vi "PID_controller_16.vi"() -> ()   [LabVIEW 2011]
panel:
  in  "Ring":u16(ring)=2 items=["A", "B", "C", "D"]
  out "do_tune":bool
  in  "Tune":bool
  out "Tune Set Point (torr)":dbl
  in  "stop":bool
  out "fit":cluster{"element":dbl, "Value":dbl}[](array[cluster])
  out "err_avg":dbl
  out "Setpoint":string
  in  "Ks":dbl
  out "dt(s)":dbl
  out "windup error":dbl
  out "tPrev":dbl
  out "target value":dbl
  out "error(t-t0)":cluster{dbl, "Value":dbl}[](array[cluster])
  out "error":dbl
  out "tStart(s)":dbl
  out "S00":dbl
  out "S10":dbl
  out "S20":dbl
  out "S11":dbl
  out "S01":dbl
  out "weight":dbl[](array[numeric])
  in  "# of points to watch":i32=60
  in  "tSmooth(s)":dbl=4.0
  out "t0":dbl
  out "error(t)":cluster{dbl, "Value":dbl}[](array[cluster])
  out "error out":errorcluster
  out "first":bool=TRUE
  out "XY Graph":T1(graph)
  out "current value":dbl
  in  "Period (s)":dbl=1.0
  out "dValue":dbl
  out "derivative":dbl
  out "integral":dbl
  out "Angle (deg)":dbl
  in  "Kd":dbl=0.4
  in  "Ki":dbl
  in  "Kp":dbl=-0.1
  out "Current P (torr)":dbl
  in  "Set Point (torr)":dbl
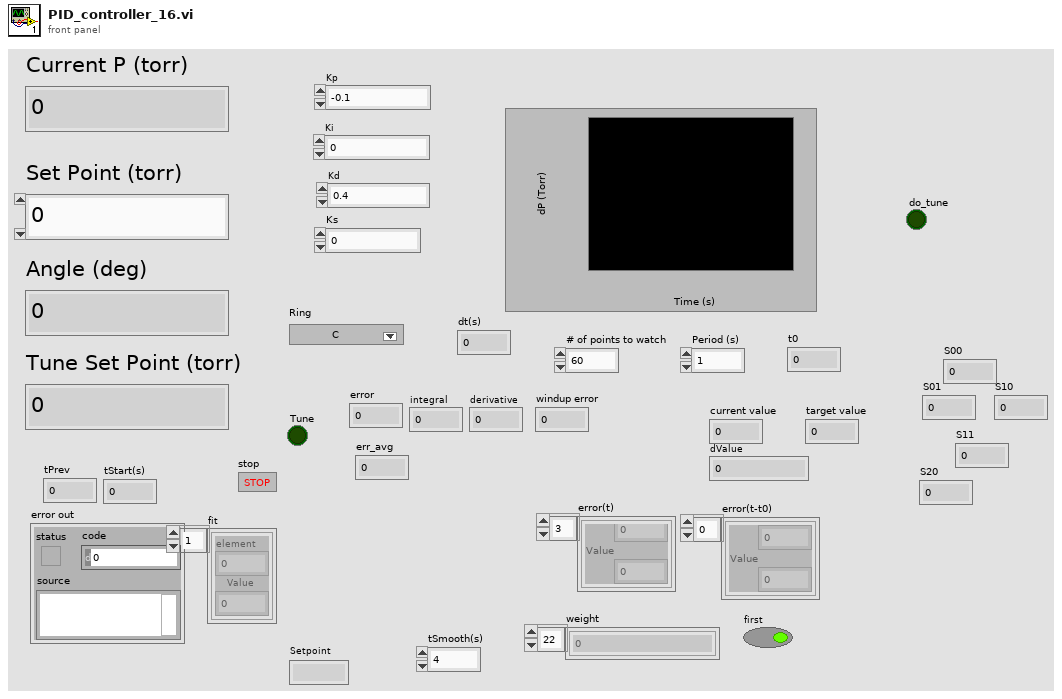
[diagram p1: front panel]
types:
  T1 = cluster{"Value":cluster{"element":dbl, "Value":dbl}[]}[]
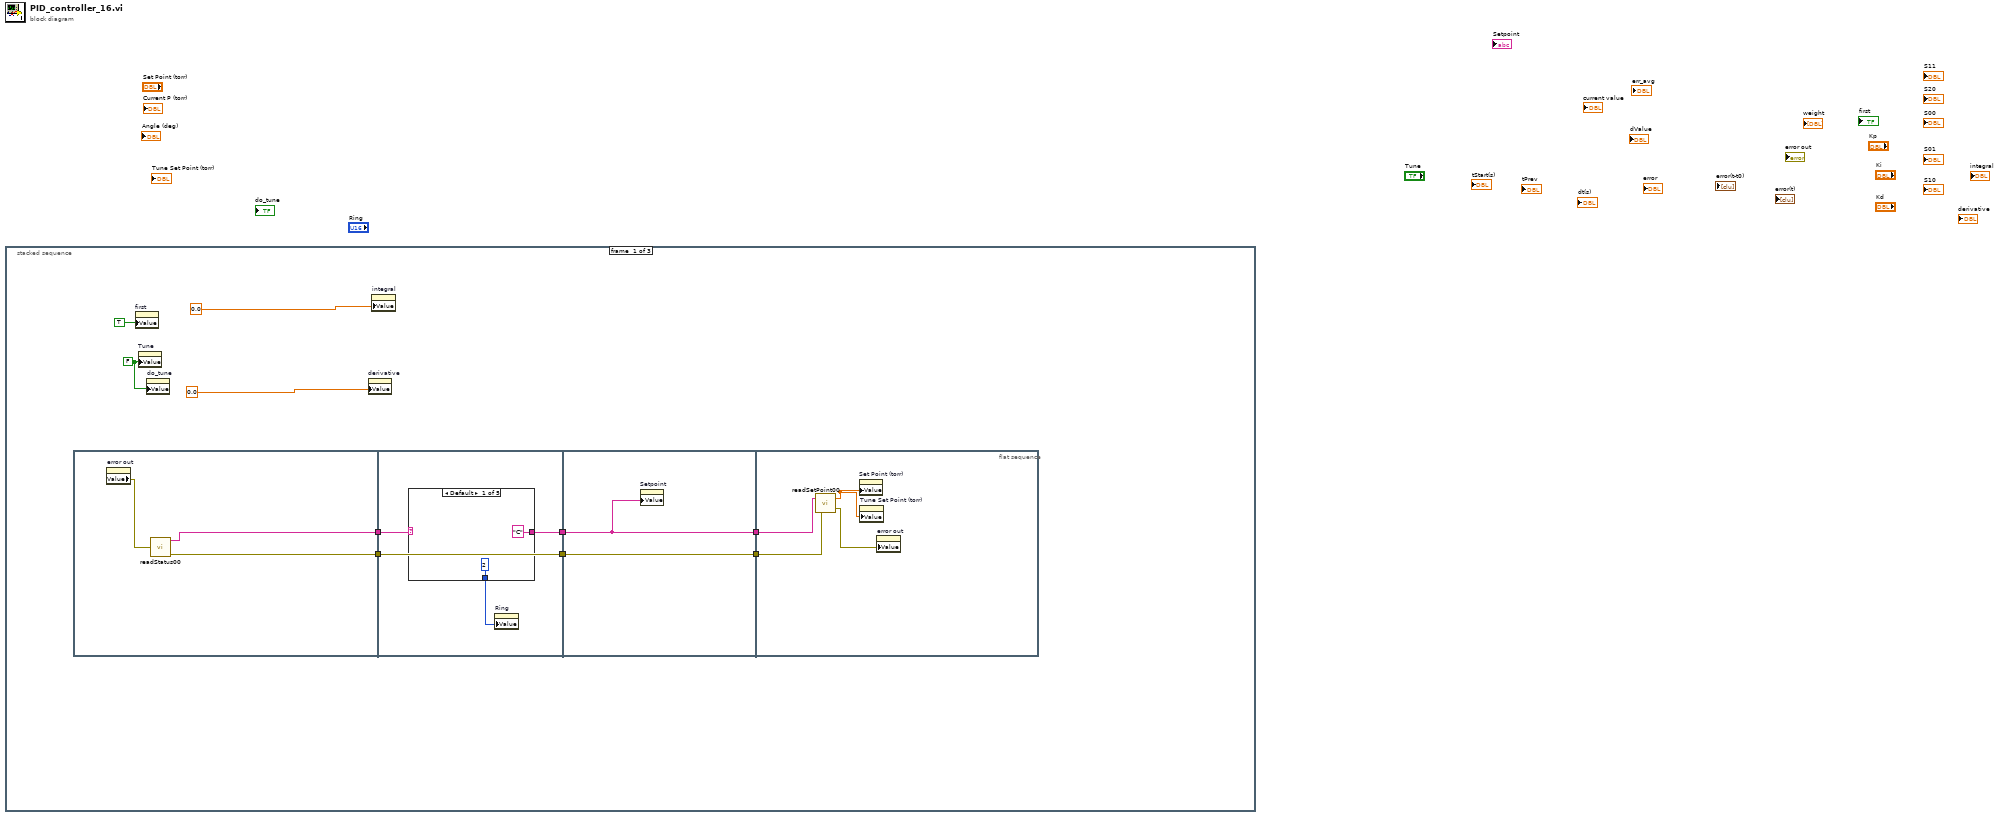
[diagram p0: block diagram]
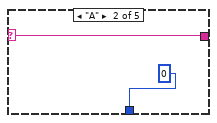
[diagram p2: hidden frame]
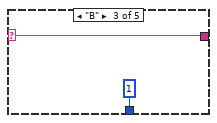
[diagram p3: hidden frame]
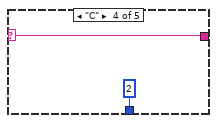
[diagram p4: hidden frame]
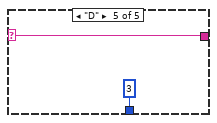
[diagram p5: hidden frame]
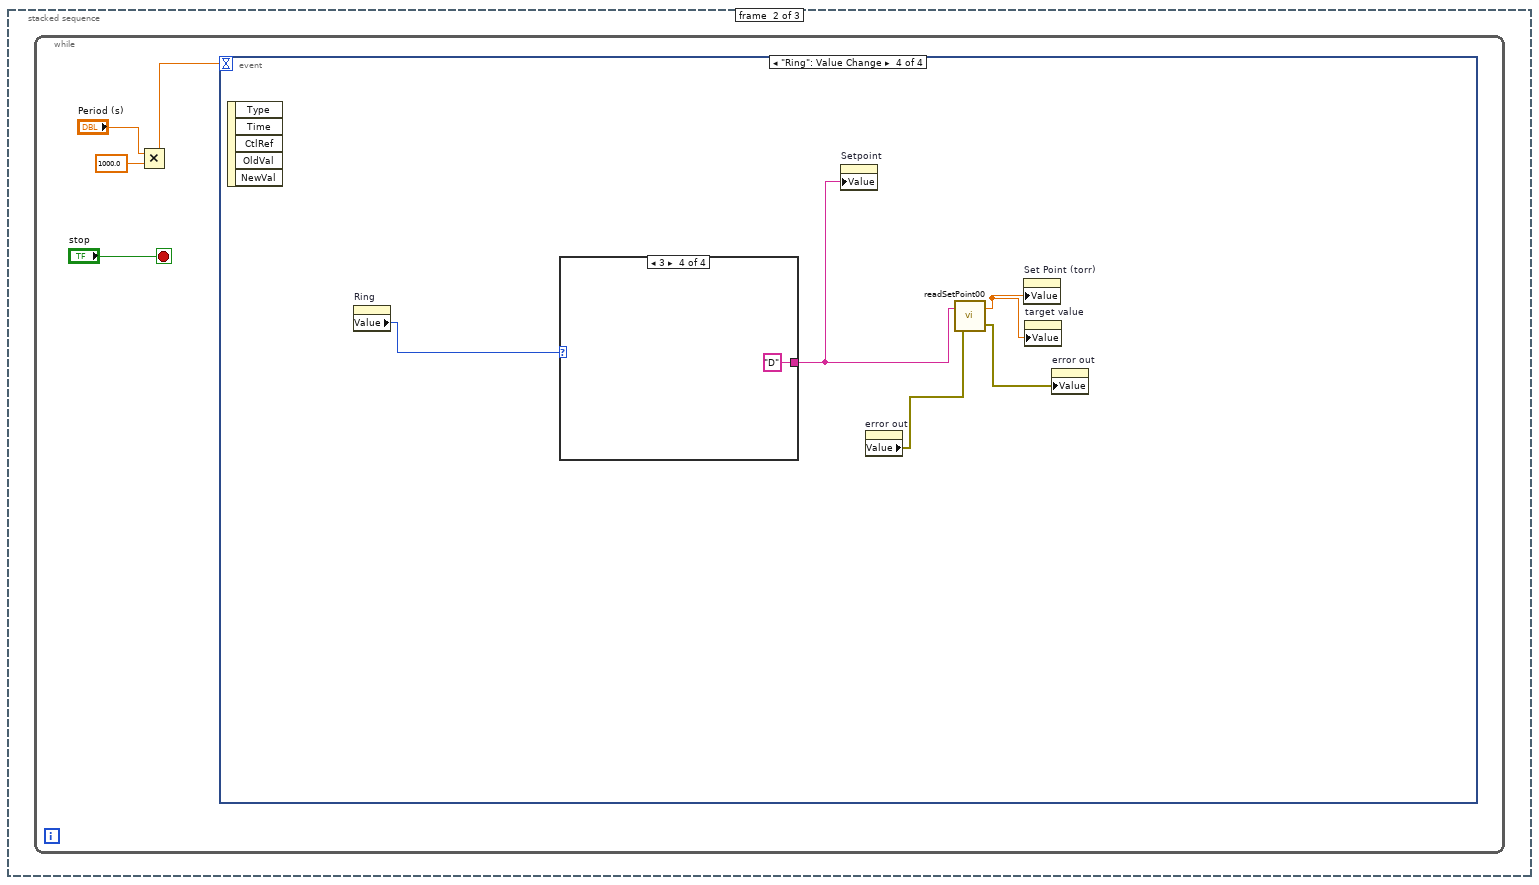
[diagram p6: hidden frame]
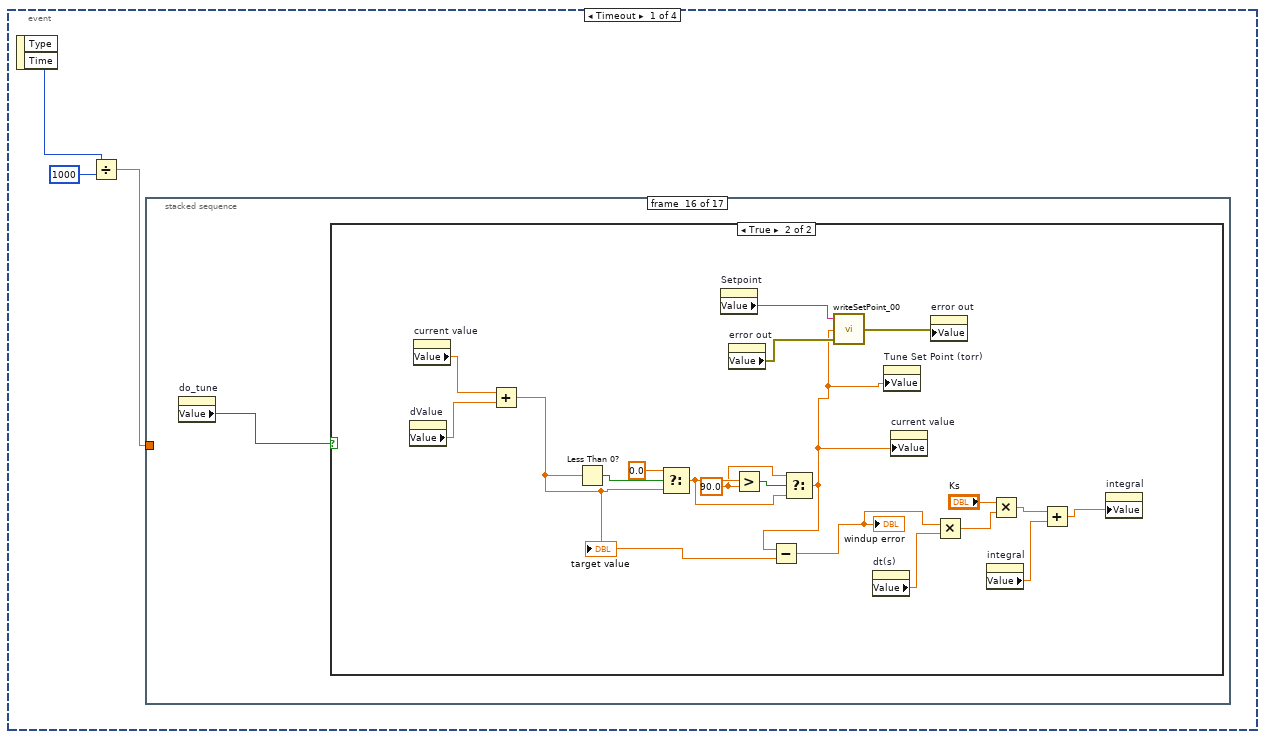
[diagram p7: hidden frame]
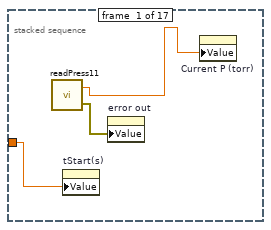
[diagram p8: hidden frame]
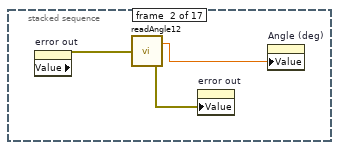
[diagram p9: hidden frame]
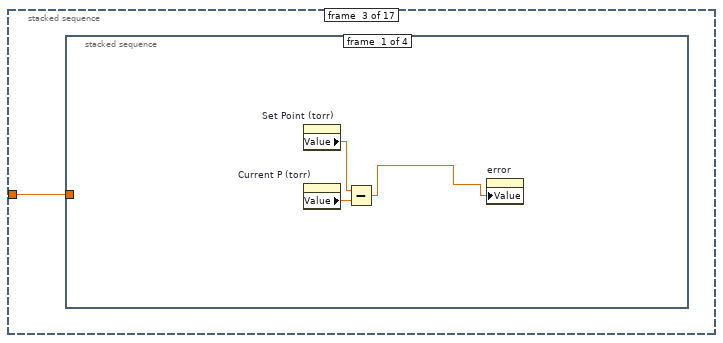
[diagram p10: hidden frame]
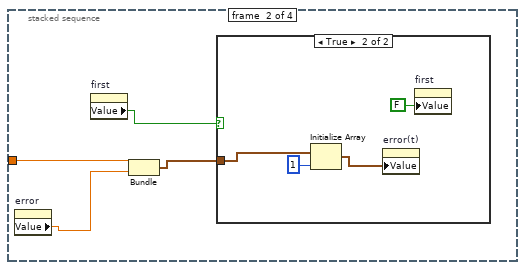
[diagram p11: hidden frame]
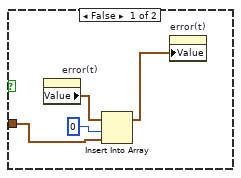
[diagram p12: hidden frame]
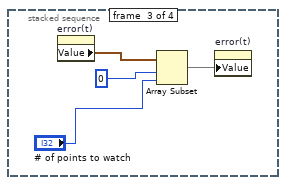
[diagram p13: hidden frame]
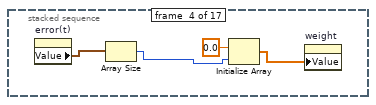
[diagram p15: hidden frame]
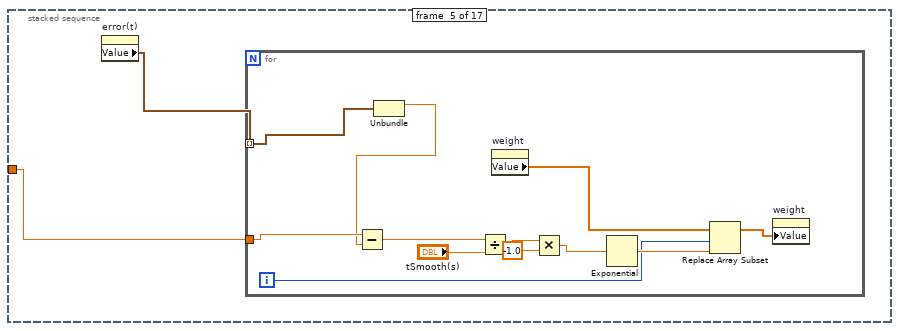
[diagram p16: hidden frame]
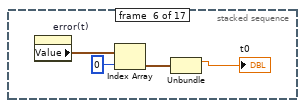
[diagram p17: hidden frame]
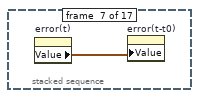
[diagram p18: hidden frame]
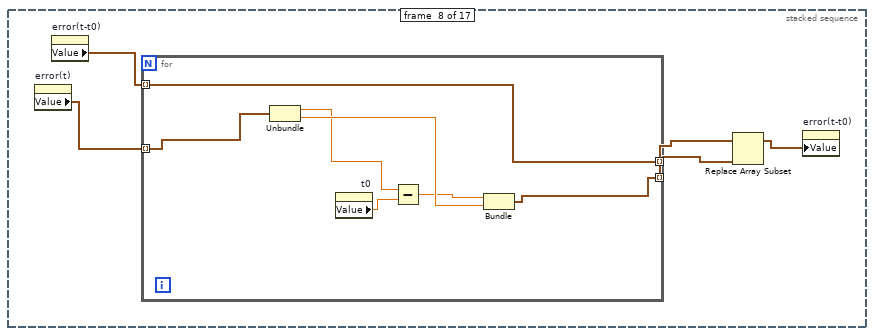
[diagram p19: hidden frame]
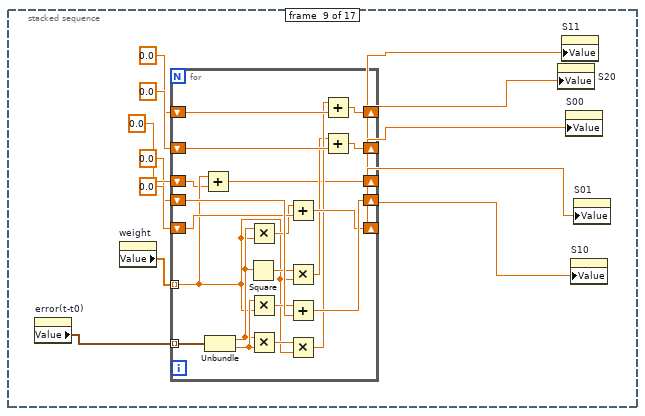
[diagram p20: hidden frame]
diagram:
  n1 = stacked-sequence {
    frame #0 {
      w7 = FALSE ("Tune")
      n2 = flat-sequence {
        tunnel: [w12] -> w6
        tunnel: [w11] -> w5
        tunnel: w6 -> [w16]
        tunnel: [w15] -> w4
        tunnel: w5 -> [w17]
        tunnel: [w17] -> w2
        tunnel: w4 -> [w28]
        tunnel: [w28] -> w3
        tunnel: w2 -> [w29]
        tunnel: [w29] -> w1
        tunnel: w3 -> [w33]
        tunnel: w1 -> [w32]
        frame #0 {
          n3 = property on="error out" class="Clust (strict)"() -> ("Value"=w13:errorcluster)  [unwired: 2 in, 2 out]
          n4 = call "readStatus00.vi"("error in"=w13) -> ("Setpoint"=w12:string, "error out"=w11:errorcluster)  [unwired: 1 out]
        }
        frame #1 {
          n5 = case shown="Default" w16 {
            selector: w16 -> [_ w21 w22 w24 w26]
            tunnel: ["C" w21 w22 w24 w26] -> w15
            tunnel: [u16 2 ("Ring") u16 0 ("Ring") u16 1 ("Ring") u16 2 ("Ring") u16 3 ("Ring")] -> w14
            frame Default {
            }
            frame "A" {
            }
            frame "B" {
            }
            frame "C" {
            }
            frame "D" {
            }
          }
          n6 = property on="Ring" class="Ring (strict)"("Value"=w14) -> ()  [unwired: 2 in, 2 out]
        }
        frame #2 {
          n7 = property on="Setpoint" class="Str"("Value"=w28) -> ()  [unwired: 2 in, 2 out]
        }
        frame #3 {
          n8 = call "readSetPoint00.vi"("error in"=w32, "Setpoint"=w33) -> ("error out"=w31:errorcluster, "P"=w30:dbl)
          n9 = property on="Set Point (torr)" class="DigNum (strict)"("Value"=w30) -> ()  [unwired: 2 in, 2 out]
          n10 = property on="Tune Set Point (torr)" class="DigNum (strict)"("Value"=w30) -> ()  [unwired: 2 in, 2 out]
          n11 = property on="error out" class="Clust (strict)"("Value"=w31) -> ()  [unwired: 2 in, 2 out]
        }
      }
      n12 = property on="first" class="Bool (strict)"("Value"=TRUE ("first")) -> ()  [unwired: 2 in, 2 out]
      n13 = property on="Tune" class="Bool (strict)"("Value"=w7) -> ()  [unwired: 2 in, 2 out]
      n14 = property on="do_tune" class="Bool (strict)"("Value"=w7) -> ()  [unwired: 2 in, 2 out]
      n15 = property on="derivative" class="DigNum (strict)"("Value"=0.0 ("derivative")) -> ()  [unwired: 2 in, 2 out]
      n16 = property on="integral" class="DigNum (strict)"("Value"=0.0 ("integral")) -> ()  [unwired: 2 in, 2 out]
    }
    frame #1 {
      n17 = while {
        stop <- "stop" stop-if-true
        n18 = Multiply(x="Period (s)", y=1000.0) -> (x*y=w35:dbl)
        n19 = event shown="[3] \"Ring\": Value Change" {
          selector: _ -> [_ _ _ _]
          dyn-events: _ -> [_ _ _ _]
          timeout: w35 -> [_ _ _ _]
          event Timeout {
            n20 = event-data() -> ("Time"=w40:u32)  [unwired: 1 in, 1 out]
            n21 = Divide(x=w40, y=u32 1000) -> (x/y=w38:dbl)
            n22 = stacked-sequence {
              tunnel: w38 -> [w41 _ w47 _ w71 _ _ _ _ _ _ _ _ _ _ _ _]
              frame #0 {
                n23 = call "readPress11.vi"() -> ("P"=w43:dbl, "error out"=w42:errorcluster)  [unwired: 1 in]
                n24 = property on="tStart(s)" class="DigNum (strict)"("Value"=w41) -> ()  [unwired: 2 in, 2 out]
                n25 = property on="error out" class="Clust (strict)"("Value"=w42) -> ()  [unwired: 2 in, 2 out]
                n26 = property on="Current P (torr)" class="DigNum (strict)"("Value"=w43) -> ()  [unwired: 2 in, 2 out]
              }
              frame #1 {
                n27 = property on="error out" class="Clust (strict)"() -> ("Value"=w45:errorcluster)  [unwired: 2 in, 2 out]
                n28 = call "readAngle12.vi"("error in"=w45) -> ("angle"=w46:dbl, "error out"=w44:errorcluster)
                n29 = property on="error out" class="Clust (strict)"("Value"=w44) -> ()  [unwired: 2 in, 2 out]
                n30 = property on="Angle (deg)" class="DigNum (strict)"("Value"=w46) -> ()  [unwired: 2 in, 2 out]
              }
              frame #2 {
                n31 = stacked-sequence {
                  tunnel: w47 -> [_ w53 _ _]
                  frame #0 {
                    n32 = property on="Set Point (torr)" class="DigNum (strict)"() -> ("Value"=w49:dbl)  [unwired: 2 in, 2 out]
                    n33 = property on="Current P (torr)" class="DigNum (strict)"() -> ("Value"=w50:dbl)  [unwired: 2 in, 2 out]
                    n34 = Subtract(x=w49, y=w50) -> (x-y=w48:dbl)
                    n35 = property on="error" class="DigNum (strict)"("Value"=w48) -> ()  [unwired: 2 in, 2 out]
                  }
                  frame #1 {
                    n36 = property on="error" class="DigNum (strict)"() -> ("Value"=w51:dbl)  [unwired: 2 in, 2 out]
                    n37 = property on="first" class="Bool (strict)"() -> ("Value"=w54:bool)  [unwired: 2 in, 2 out]
                    n38 = Bundle(w53, "Value"=w51) -> (w52:cluster{dbl, "Value":dbl})  [unwired: 1 in]
                    n39 = case shown="True" w54 {
                      tunnel: w52 -> [w56 w61]
                      frame False {
                        n40 = property on="error(t)" class="Arr (strict)"() -> ("Value"=w57:cluster{dbl, "Value":dbl}[])  [unwired: 2 in, 2 out]
                        n41 = Insert Into Array(array=w57, index=0, new element=w56) -> (w55:cluster{dbl, "Value":dbl}[])
                        n42 = property on="error(t)" class="Arr (strict)"("Value"=w55) -> ()  [unwired: 2 in, 2 out]
                      }
                      frame True {
                        n43 = Initialize Array(w61, 1 ("dimension size")) -> (w59:cluster{dbl, "Value":dbl}[])
                        n44 = property on="error(t)" class="Arr (strict)"("Value"=w59) -> ()  [unwired: 2 in, 2 out]
                        n45 = property on="first" class="Bool (strict)"("Value"=FALSE ("first")) -> ()  [unwired: 2 in, 2 out]
                      }
                    }
                  }
                  frame #2 {
                    n46 = property on="error(t)" class="Arr (strict)"() -> ("Value"=w64:cluster{dbl, "Value":dbl}[])  [unwired: 2 in, 2 out]
                    n47 = Array Subset(array=w64, index=0, length="# of points to watch") -> (w66:cluster{dbl, "Value":dbl}[])
                    n48 = property on="error(t)" class="Arr (strict)"("Value"=w66) -> ()  [unwired: 2 in, 2 out]
                  }
                  frame #3 {
                  }
                }
              }
              frame #3 {
                n49 = property on="error(t)" class="Arr (strict)"() -> ("Value"=w67:cluster{dbl, "Value":dbl}[])  [unwired: 2 in, 2 out]
                n50 = Array Size(array=w67) -> (size(s)=w69:i32)
                n51 = Initialize Array(0.0 ("element"), w69) -> (w70:dbl[])
                n52 = property on="weight" class="Arr (strict)"("Value"=w70) -> ()  [unwired: 2 in, 2 out]
              }
              frame #4 {
                n53 = property on="error(t)" class="Arr (strict)"() -> ("Value"=w72:cluster{dbl, "Value":dbl}[])  [unwired: 2 in, 2 out]
                n54 = for {
                  tunnel: w72 -> [w84] mode=indexing
                  tunnel: w71 -> [w83]
                  i -> [w79]
                  n55 = Unbundle(w84) -> (w82:dbl)  [unwired: 1 out]
                  n56 = Subtract(x=w83, y=w82) -> (x-y=w77:dbl)
                  n57 = Divide(x=w77, y="tSmooth(s)") -> (x/y=w75:dbl)
                  n58 = property on="weight" class="Arr (strict)"() -> ("Value"=w80:dbl[])  [unwired: 2 in, 2 out]
                  n59 = Multiply(x=w75, y=-1.0) -> (x*y=w73:dbl)
                  n60 = Exponential(1:w73) -> (0:w81:dbl)
                  n61 = Replace Array Subset(array=w80, new element=w81, index=w79) -> (w78:dbl[])
                  n62 = property on="weight" class="Arr (strict)"("Value"=w78) -> ()  [unwired: 2 in, 2 out]
                }
              }
              frame #5 {
                n63 = property on="error(t)" class="Arr (strict)"() -> ("Value"=w85:cluster{dbl, "Value":dbl}[])  [unwired: 2 in, 2 out]
                n64 = Index Array(array=w85, index=0) -> (element=w87:cluster{dbl, "Value":dbl})
                n65 = Unbundle(w87) -> (→"t0":dbl)  [unwired: 1 out]
              }
              frame #6 {
                n66 = property on="error(t)" class="Arr (strict)"() -> ("Value"=w89:cluster{dbl, "Value":dbl}[])  [unwired: 2 in, 2 out]
                n67 = property on="error(t-t0)" class="Arr (strict)"("Value"=w89) -> ()  [unwired: 2 in, 2 out]
              }
              frame #7 {
                n68 = property on="error(t)" class="Arr (strict)"() -> ("Value"=w90:cluster{dbl, "Value":dbl}[])  [unwired: 2 in, 2 out]
                n69 = property on="error(t-t0)" class="Arr (strict)"() -> ("Value"=w92:cluster{dbl, "Value":dbl}[])  [unwired: 2 in, 2 out]
                n70 = for {
                  tunnel: w90 -> [w97] mode=indexing
                  tunnel: [w96] -> w91 mode=indexing
                  tunnel: w92 -> [w95] mode=indexing
                  tunnel: [w95] -> w93 mode=indexing
                  n71 = Unbundle(w97) -> (w98:dbl, "Value"=w100:dbl)
                  n72 = property on="t0" class="DigNum (strict)"() -> ("Value"=w101:dbl)  [unwired: 2 in, 2 out]
                  n73 = Subtract(x=w98, y=w101) -> (x-y=w99:dbl)
                  n74 = Bundle(w99, "Value"=w100) -> (w96:cluster{dbl, "Value":dbl})  [unwired: 1 in]
                }
                n75 = Replace Array Subset(array=w93, new element=w91) -> (w94:cluster{dbl, "Value":dbl}[])  [unwired: 1 in]
                n76 = property on="error(t-t0)" class="Arr (strict)"("Value"=w94) -> ()  [unwired: 2 in, 2 out]
              }
              frame #8 {
                n77 = property on="error(t-t0)" class="Arr (strict)"() -> ("Value"=w113:cluster{dbl, "Value":dbl}[])  [unwired: 2 in, 2 out]
                n78 = property on="weight" class="Arr (strict)"() -> ("Value"=w106:dbl[])  [unwired: 2 in, 2 out]
                n79 = for {
                  tunnel: w113 -> [w129] mode=indexing
                  shift-right: [w130] -> w111
                  shift-left: 0.0 -> [w133]
                  shift-right: [w126] -> w108
                  shift-left: 0.0 -> [w132]
                  shift-right: [w125] -> w109
                  shift-left: 0.0 -> [w131]
                  shift-right: [w127] -> w112
                  shift-left: 0.0 -> [w128]
                  tunnel: w106 -> [w116] mode=indexing
                  shift-right: [w114] -> w110
                  shift-left: 0.0 -> [w115]
                  n80 = Add(x=w116, y=w115) -> (x+y=w114:dbl)
                  n81 = Unbundle(w129) -> (w118:dbl, "Value"=w124:dbl)
                  n82 = Square(x=w118) -> (x^2=w120:dbl)
                  n83 = Multiply(x=w118, y=w116) -> (x*y=w117:dbl)
                  n84 = Multiply(x=w124, y=w116) -> (x*y=w123:dbl)
                  n85 = Multiply(x=w118, y=w124) -> (x*y=w122:dbl)
                  n86 = Add(x=w117, y=w128) -> (x+y=w127:dbl)
                  n87 = Multiply(x=w120, y=w116) -> (x*y=w119:dbl)
                  n88 = Add(x=w123, y=w133) -> (x+y=w130:dbl)
                  n89 = Multiply(x=w122, y=w116) -> (x*y=w121:dbl)
                  n90 = Add(x=w121, y=w132) -> (x+y=w126:dbl)
                  n91 = Add(x=w119, y=w131) -> (x+y=w125:dbl)
                }
                n92 = property on="S20" class="DigNum (strict)"("Value"=w109) -> ()  [unwired: 2 in, 2 out]
                n93 = property on="S11" class="DigNum (strict)"("Value"=w108) -> ()  [unwired: 2 in, 2 out]
                n94 = property on="S00" class="DigNum (strict)"("Value"=w110) -> ()  [unwired: 2 in, 2 out]
                n95 = property on="S10" class="DigNum (strict)"("Value"=w112) -> ()  [unwired: 2 in, 2 out]
                n96 = property on="S01" class="DigNum (strict)"("Value"=w111) -> ()  [unwired: 2 in, 2 out]
              }
              frame #9 {
                n97 = property on="S00" class="DigNum (strict)"() -> ("Value"=w135:dbl)  [unwired: 2 in, 2 out]
                n98 = Greater Than 0?(x=w135) -> (x > 0?=w134:bool)
                n99 = case shown="True" w134 {
                  tunnel: w135 -> [_ w144]
                  frame False {
                    n100 = property on="derivative" class="DigNum (strict)"("Value"=0.0 ("derivative")) -> ()  [unwired: 2 in, 2 out]
                  }
                  frame True {
                    n101 = property on="S11" class="DigNum (strict)"() -> ("Value"=w146:dbl)  [unwired: 2 in, 2 out]
                    n102 = property on="S20" class="DigNum (strict)"() -> ("Value"=w145:dbl)  [unwired: 2 in, 2 out]
                    n103 = property on="S01" class="DigNum (strict)"() -> ("Value"=w143:dbl)  [unwired: 2 in, 2 out]
                    n104 = property on="S10" class="DigNum (strict)"() -> ("Value"=w147:dbl)  [unwired: 2 in, 2 out]
                    n105 = Multiply(x=w144, y=w146) -> (x*y=w152:dbl)
                    n106 = Multiply(x=w144, y=w145) -> (x*y=w150:dbl)
                    n107 = Multiply(x=w143, y=w147) -> (x*y=w151:dbl)
                    n108 = Square(x=w147) -> (x^2=w149:dbl)
                    n109 = Subtract(x=w152, y=w151) -> (x-y=w148:dbl)
                    n110 = Subtract(x=w150, y=w149) -> (x-y=w142:dbl)
                    n111 = Divide(x=w148, y=w142) -> (x/y=w138:dbl)
                    n112 = Greater?(x=w142, y=1e-07) -> (0:w140:bool)
                    n113 = Select(t=w138, s=w140, f=0.0) -> (s? t:f=w139:dbl)
                    n114 = property on="derivative" class="DigNum (strict)"("Value"=w139) -> ()  [unwired: 2 in, 2 out]
                  }
                }
              }
              frame #10 {
                n115 = property on="S00" class="DigNum (strict)"() -> ("Value"=w154:dbl)  [unwired: 2 in, 2 out]
                n116 = Greater Than 0?(x=w154) -> (x > 0?=w153:bool)
                n117 = case shown="True" w153 {
                  tunnel: w154 -> [_ w157]
                  frame False {
                    n118 = property on="err_avg" class="DigNum (strict)"("Value"=0.0 ("Pavg")) -> ()  [unwired: 2 in, 2 out]
                  }
                  frame True {
                    n119 = property on="S01" class="DigNum (strict)"() -> ("Value"=w158:dbl)  [unwired: 2 in, 2 out]
                    n120 = property on="S20" class="DigNum (strict)"() -> ("Value"=w161:dbl)  [unwired: 2 in, 2 out]
                    n121 = property on="S11" class="DigNum (strict)"() -> ("Value"=w159:dbl)  [unwired: 2 in, 2 out]
                    n122 = property on="S11" class="DigNum (strict)"() -> ("Value"=w160:dbl)  [unwired: 2 in, 2 out]
                    n123 = Multiply(x=w158, y=w161) -> (x*y=w166:dbl)
                    n124 = Multiply(x=w157, y=w161) -> (x*y=w163:dbl)
                    n125 = Multiply(x=w160, y=w159) -> (x*y=w167:dbl)
                    n126 = Square(x=w160) -> (x^2=w164:dbl)
                    n127 = Subtract(x=w166, y=w167) -> (x-y=w162:dbl)
                    n128 = Subtract(x=w163, y=w164) -> (x-y=w165:dbl)
                    n129 = Divide(x=w162, y=w165) -> (x/y=w156:dbl)
                    n130 = property on="err_avg" class="DigNum (strict)"("Value"=w156) -> ()  [unwired: 2 in, 2 out]
                  }
                }
              }
              frame #11 {
                n131 = property on="tStart(s)" class="DigNum (strict)"() -> ("Value"=w168:dbl)  [unwired: 2 in, 2 out]
                n132 = property on="tPrev" class="DigNum (strict)"("Value"=w168) -> ()  [unwired: 2 in, 2 out]
              }
              frame #12 {
                n133 = property on="error(t-t0)" class="Arr (strict)"() -> ("Value"=w169:cluster{dbl, "Value":dbl}[])  [unwired: 2 in, 2 out]
                n134 = Array Size(array=w169) -> (size(s)=w170:i32)
                n135 = Greater?(x=w170, y=1) -> (0:w172:bool)
                n136 = case shown="True" w172 {
                  frame False {
                  }
                  frame True {
                    n137 = property on="error(t-t0)" class="Arr (strict)"() -> ("Value"=w176:cluster{dbl, "Value":dbl}[])  [unwired: 2 in, 2 out]
                    n138 = Array Size(array=w176) -> (size(s)=w186:i32)
                    n139 = Index Array(array=w176, index=0) -> (element=w184:cluster{dbl, "Value":dbl})
                    n140 = Unbundle(w184) -> (w179:dbl)  [unwired: 1 out]
                    n141 = Decrement(x=w186) -> (x-1=w185:i32)
                    n142 = Index Array(array=w176, index=w185) -> (element=w183:cluster{dbl, "Value":dbl})
                    n143 = Unbundle(w183) -> (w177:dbl)  [unwired: 1 out]
                    n144 = property on="derivative" class="DigNum (strict)"() -> ("Value"=w182:dbl)  [unwired: 2 in, 2 out]
                    n145 = property on="error" class="DigNum (strict)"() -> ("Value"=w180:dbl)  [unwired: 2 in, 2 out]
                    n146 = Multiply(x=w177, y=w182) -> (x*y=w181:dbl)
                    n147 = Add(x=w180, y=w181) -> (x+y=w178:dbl)
                    n148 = Bundle(w179, "Value"=w180) -> (w175:cluster{dbl, "Value":dbl})  [unwired: 1 in]
                    n149 = Bundle(w177, w178) -> (w174:cluster{dbl, dbl})  [unwired: 1 in]
                    n150 = Build Array(w175, w174) -> (→"fit":cluster{dbl, "Value":dbl}[])
                  }
                }
              }
              frame #13 {
                n151 = property on="error" class="DigNum (strict)"() -> ("Value"=w190:dbl)  [unwired: 2 in, 2 out]
                n152 = property on="tPrev" class="DigNum (strict)"() -> ("Value"=w189:dbl)  [unwired: 2 in, 2 out]
                n153 = property on="tStart(s)" class="DigNum (strict)"() -> ("Value"=w188:dbl)  [unwired: 2 in, 2 out]
                n154 = Subtract(x=w188, y=w189) -> (x-y=w194:dbl)
                n155 = property on="dt(s)" class="DigNum (strict)"("Value"=w194) -> ()  [unwired: 2 in, 2 out]
                n156 = property on="integral" class="DigNum (strict)"() -> ("Value"=w192:dbl)  [unwired: 2 in, 2 out]
                n157 = Multiply(x=w190, y=w194) -> (x*y=w191:dbl)
                n158 = Add(x=w191, y=w192) -> (x+y=w193:dbl)
                n159 = property on="integral" class="DigNum (strict)"("Value"=w193) -> ()  [unwired: 2 in, 2 out]
              }
              frame #14 {
                n160 = property on="error" class="DigNum (strict)"() -> ("Value"=w205:dbl)  [unwired: 2 in, 2 out]
                n161 = property on="Kp" class="DigNum (strict)"() -> ("Value"=w195:dbl)  [unwired: 2 in, 2 out]
                n162 = property on="integral" class="DigNum (strict)"() -> ("Value"=w197:dbl)  [unwired: 2 in, 2 out]
                n163 = property on="derivative" class="DigNum (strict)"() -> ("Value"=w199:dbl)  [unwired: 2 in, 2 out]
                n164 = property on="Ki" class="DigNum (strict)"() -> ("Value"=w196:dbl)  [unwired: 2 in, 2 out]
                n165 = property on="Kd" class="DigNum (strict)"() -> ("Value"=w198:dbl)  [unwired: 2 in, 2 out]
                n166 = Multiply(x=w198, y=w199) -> (x*y=w202:dbl)
                n167 = Multiply(x=w196, y=w197) -> (x*y=w201:dbl)
                n168 = Multiply(x=w195, y=w205) -> (x*y=w200:dbl)
                n169 = Add(x=w200, y=w201) -> (x+y=w203:dbl)
                n170 = Add(x=w203, y=w202) -> (x+y=w204:dbl)
                n171 = property on="dValue" class="DigNum (strict)"("Value"=w204) -> ()  [unwired: 2 in, 2 out]
              }
              frame #15 {
                n172 = property on="do_tune" class="Bool (strict)"() -> ("Value"=w206:bool)  [unwired: 2 in, 2 out]
                n173 = case shown="True" w206 {
                  frame False {
                  }
                  frame True {
                    w217 = 90.0 ("y")
                    n174 = property on="dValue" class="DigNum (strict)"() -> ("Value"=w224:dbl)  [unwired: 2 in, 2 out]
                    n175 = property on="current value" class="DigNum (strict)"() -> ("Value"=w225:dbl)  [unwired: 2 in, 2 out]
                    n176 = Add(x=w225, y=w224) -> (x+y=w209:dbl)
                    "target value" <- w209
                    n177 = Less Than 0?(x=w209) -> (x < 0?=w221:bool)
                    n178 = Select(t=0.0, s=w221, f=w209) -> (s? t:f=w218:dbl)
                    n179 = property on="Setpoint" class="Str"() -> ("Value"=w208:string)  [unwired: 2 in, 2 out]
                    n180 = property on="error out" class="Clust (strict)"() -> ("Value"=w223:errorcluster)  [unwired: 2 in, 2 out]
                    n181 = Greater?(x=w218, y=w217) -> (0:w219:bool)
                    n182 = Select(t=w217, s=w219, f=w218) -> (s? t:f=w207:dbl)
                    n183 = Subtract(x=w207, y=w209) -> (x-y=w216:dbl)
                    "windup error" <- w216
                    n184 = call "writeSetPoint_00.vi"("error in"=w223, "P (Torr)"=w207, "Setpoint"=w208) -> ("error out"=w222:errorcluster)
                    n185 = property on="dt(s)" class="DigNum (strict)"() -> ("Value"=w215:dbl)  [unwired: 2 in, 2 out]
                    n186 = property on="Tune Set Point (torr)" class="DigNum (strict)"("Value"=w207) -> ()  [unwired: 2 in, 2 out]
                    n187 = property on="current value" class="DigNum (strict)"("Value"=w207) -> ()  [unwired: 2 in, 2 out]
                    n188 = property on="error out" class="Clust (strict)"("Value"=w222) -> ()  [unwired: 2 in, 2 out]
                    n189 = Multiply(x=w216, y=w215) -> (x*y=w214:dbl)
                    n190 = property on="integral" class="DigNum (strict)"() -> ("Value"=w211:dbl)  [unwired: 2 in, 2 out]
                    n191 = Multiply(x="Ks", y=w214) -> (x*y=w212:dbl)
                    n192 = Add(x=w212, y=w211) -> (x+y=w210:dbl)
                    n193 = property on="integral" class="DigNum (strict)"("Value"=w210) -> ()  [unwired: 2 in, 2 out]
                  }
                }
              }
              frame #16 {
                n194 = property on="fit" class="Arr (strict)"() -> ("Value"=w228:cluster{"element":dbl, "Value":dbl}[])  [unwired: 2 in, 2 out]
                n195 = property on="error(t-t0)" class="Arr (strict)"() -> ("Value"=w227:cluster{dbl, "Value":dbl}[])  [unwired: 2 in, 2 out]
                n196 = Build Cluster Array(w227, w228) -> (→"XY Graph":T1)
              }
            }
          }
          event "Tune": Value Change {
            n197 = event-data() -> ()  [unwired: 1 in, 5 out]
            n198 = property on="Tune" class="Bool (strict)"() -> ("Value"=w229:bool)  [unwired: 2 in, 2 out]
            n199 = property on="do_tune" class="Bool (strict)"("Value"=w229) -> ()  [unwired: 2 in, 2 out]
            n200 = case shown="True" w229 {
              frame False {
                n201 = property on="Set Point (torr)" class="DigNum (strict)"() -> ("Value"=w232:dbl)  [unwired: 2 in, 2 out]
                n202 = property on="Setpoint" class="Str"() -> ("Value"=w233:string)  [unwired: 2 in, 2 out]
                n203 = property on="error out" class="Clust (strict)"() -> ("Value"=w231:errorcluster)  [unwired: 2 in, 2 out]
                n204 = call "writeSetPoint_00.vi"("error in"=w231, "P (Torr)"=w232, "Setpoint"=w233) -> ("error out"=w230:errorcluster)
                n205 = property on="error out" class="Clust (strict)"("Value"=w230) -> ()  [unwired: 2 in, 2 out]
              }
              frame True {
                n206 = property on="error out" class="Clust (strict)"() -> ("Value"=w236:errorcluster)  [unwired: 2 in, 2 out]
                n207 = property on="Setpoint" class="Str"() -> ("Value"=w235:string)  [unwired: 2 in, 2 out]
                n208 = call "readSetPoint00.vi"("error in"=w236, "Setpoint"=w235) -> ("error out"=w237:errorcluster, "P"=w234:dbl)
                n209 = property on="Tune Set Point (torr)" class="DigNum (strict)"("Value"=w234) -> ()  [unwired: 2 in, 2 out]
                n210 = property on="Set Point (torr)" class="DigNum (strict)"("Value"=w234) -> ()  [unwired: 2 in, 2 out]
                n211 = property on="error out" class="Clust (strict)"("Value"=w237) -> ()  [unwired: 2 in, 2 out]
                n212 = property on="current value" class="DigNum (strict)"("Value"=w234) -> ()  [unwired: 2 in, 2 out]
              }
            }
          }
          event "Set Point (torr)": Value Change {
            n213 = event-data() -> ()  [unwired: 1 in, 5 out]
            n214 = property on="Set Point (torr)" class="DigNum (strict)"() -> ("Value"=w240:dbl)  [unwired: 2 in, 2 out]
            n215 = property on="Setpoint" class="Str"() -> ("Value"=w241:string)  [unwired: 2 in, 2 out]
            n216 = property on="error out" class="Clust (strict)"() -> ("Value"=w239:errorcluster)  [unwired: 2 in, 2 out]
            n217 = call "writeSetPoint_00.vi"("error in"=w239, "P (Torr)"=w240, "Setpoint"=w241) -> ("error out"=w238:errorcluster)
            n218 = property on="error out" class="Clust (strict)"("Value"=w238) -> ()  [unwired: 2 in, 2 out]
          }
          event "Ring": Value Change {
            n219 = event-data() -> ()  [unwired: 1 in, 5 out]
            n220 = property on="Ring" class="Ring (strict)"() -> ("Value"=w246:u16)  [unwired: 2 in, 2 out]
            n221 = case shown="3" w246 {
              tunnel: ["A" "B" "C" "D"] -> w242
              frame 0, Default {
              }
              frame 1 {
              }
              frame 2 {
              }
              frame 3 {
              }
            }
            n222 = property on="Setpoint" class="Str"("Value"=w242) -> ()  [unwired: 2 in, 2 out]
            n223 = property on="error out" class="Clust (strict)"() -> ("Value"=w243:errorcluster)  [unwired: 2 in, 2 out]
            n224 = call "readSetPoint00.vi"("error in"=w243, "Setpoint"=w242) -> ("error out"=w244:errorcluster, "P"=w245:dbl)
            n225 = property on="Set Point (torr)" class="DigNum (strict)"("Value"=w245) -> ()  [unwired: 2 in, 2 out]
            n226 = property on="target value" class="DigNum (strict)"("Value"=w245) -> ()  [unwired: 2 in, 2 out]
            n227 = property on="error out" class="Clust (strict)"("Value"=w244) -> ()  [unwired: 2 in, 2 out]
          }
        }
      }
    }
    frame #2 {
      n228 = disable-structure shown="Disabled" {
        frame Disabled {
          n229 = flat-sequence {
            frame #0 {
              n230 = call "WriteAdaptorr03.vi"("string to write"="D5") -> ()  [unwired: 1 in, 1 out]
            }
            frame #1 {
              n231 = property on="Setpoint" class="Str"() -> ("Value"=w253:string)  [unwired: 2 in, 2 out]
              n232 = Concatenate Strings("Press ", w253, " on AdapTorr") -> (w252:string)
              n233 = One Button Dialog(message=w252) -> ()  [unwired: 1 in, 1 out]
            }
          }
        }
        frame Enabled {
        }
      }
    }
  }
